vi "Read Manual Range.vi"(8 "error in (no error)":errorcluster, 11 "DMM in":refnum<class "DMM.lvclass">) -> (0 "error out":errorcluster, 2 "Manual Range":dbl, 3 "DMM out":refnum<class "DMM.lvclass">)   [LabVIEW 2018, in "DMM.lvlib" / "DMM.lvclass"]
uses:
  DMM.lvclass
  DMM.lvclass/DMM.ctl
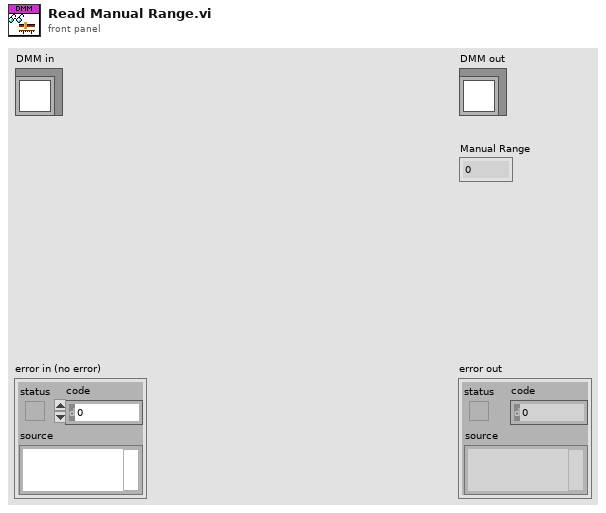
[diagram p1: front panel]
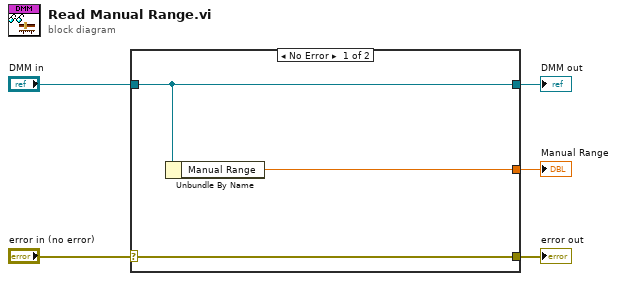
[diagram p0: block diagram]
diagram:
  n1 = case shown="No Error" "error in (no error)" {
    selector: "error in (no error)" -> [w8 w9]
    tunnel: [w8 w9] -> w4
    tunnel: [w7 w10] -> w2
    tunnel: "DMM in" -> [w7 w10]
    tunnel: [w6 _] -> w1
    frame No Error {
      n2 = Unbundle By Name(w7) -> ("Manual Range"=w6:dbl)
    }
    frame Error {
    }
  }
  "error out" <- w4
  "DMM out" <- w2
  "Manual Range" <- w1
